vi "Send SCPI Strings.vi"(0 "Resource In":refnum<visa-resource-name>, 1 "Check For SCPI Errors? (T)":bool=TRUE, 5 "SCPI Strings (no term char)":string[](array[string]), 7 "Term Char (0xA)":u8=10 format="%02x", 9 "Num Bytes To Read (256)":u32=256, 11 "error in (no error)":errorcluster, 14 "Trim End Whitespace? (T)":bool=TRUE) -> (4 "Resource Out (dupl)":refnum<visa-resource-name>, 6 "Query Responses":string[](array[string]), 8 "Num Strings Sent":i32, 15 "error out":errorcluster)   [LabVIEW 2009, in "Keithley 622x.lvlib"]
uses:
  Keithley 622x.lvlib
  <vilib>/Utility/error.llb/whitespace.ctl
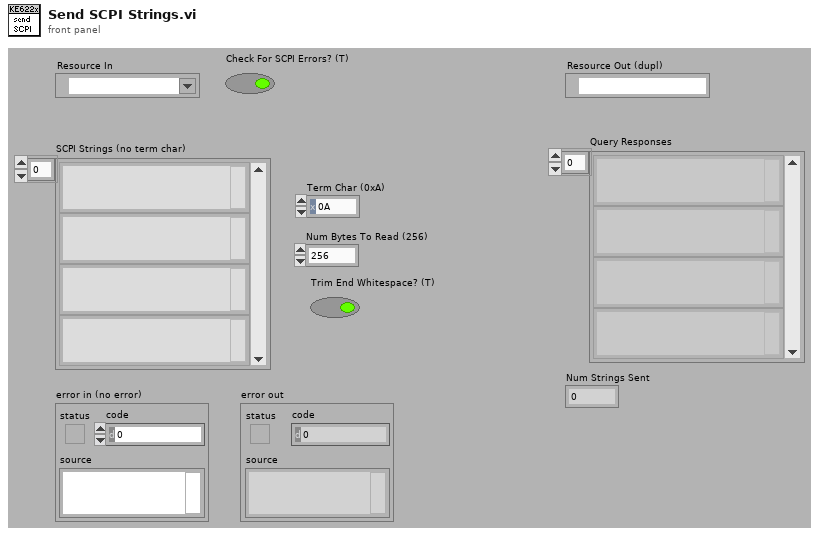
[diagram p1: front panel]
types:
  T1 = typedef "whitespace.ctl" = u16
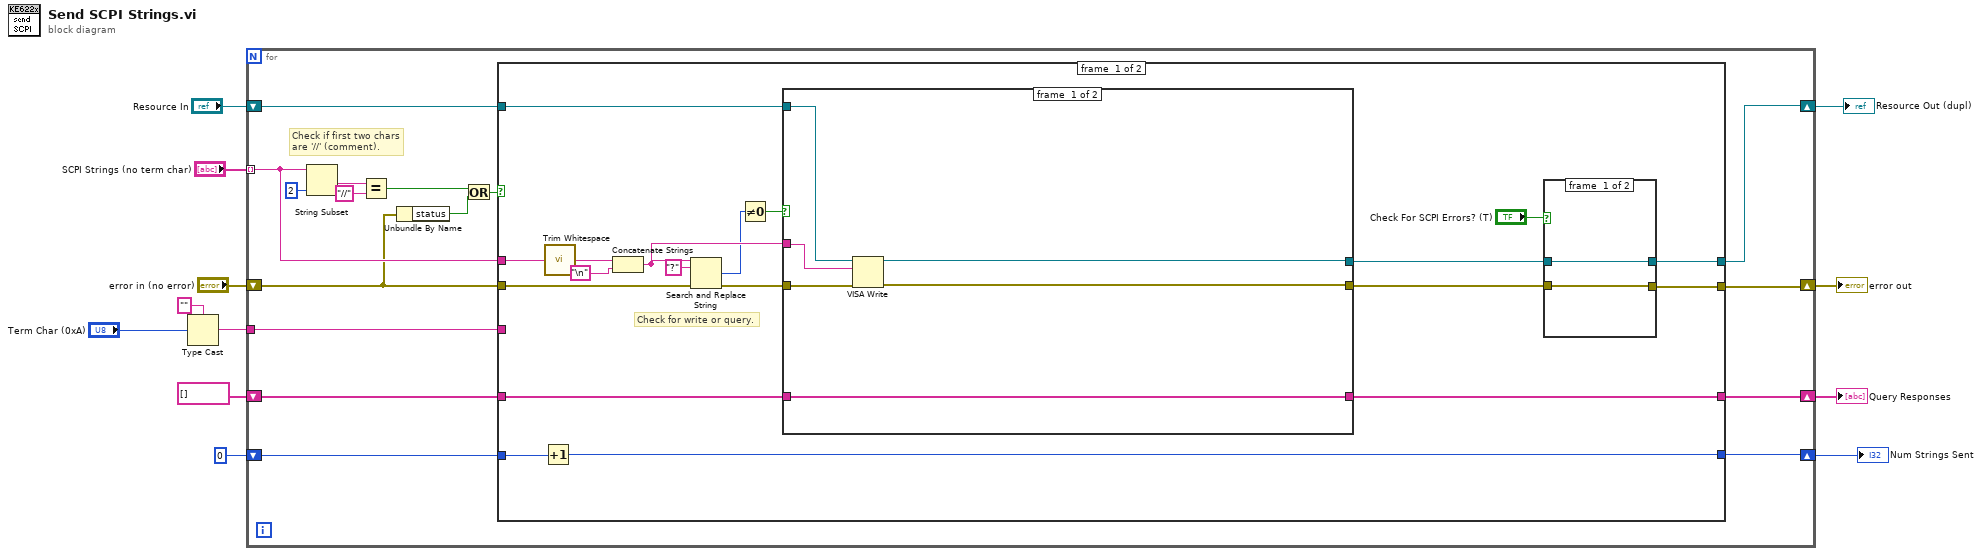
[diagram p0: block diagram]
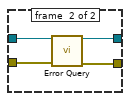
[diagram p2: hidden frame]
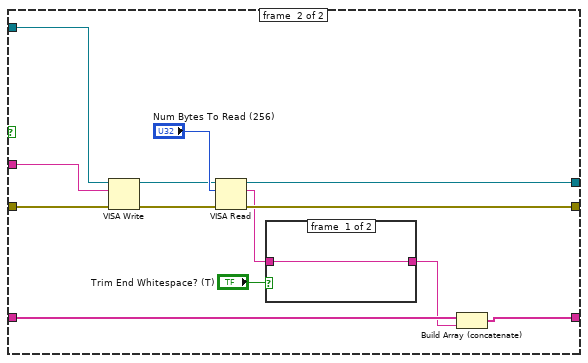
[diagram p3: hidden frame]
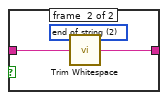
[diagram p4: hidden frame]
diagram:
  n1 = Type Cast(type="", x="Term Char (0xA)") -> (*(type *) &x=w1:string)
  n2 = for {
    tunnel: "SCPI Strings (no term char)" -> [w24] mode=indexing
    shift-right: [w19] -> w6
    shift-left: "error in (no error)" -> [w17]
    shift-right: [w18] -> w5
    shift-left: "Resource In" -> [w23]
    tunnel: w1 -> [w22]
    shift-right: [w20] -> w4
    shift-left: string[] [] -> [w21]
    shift-right: [w13] -> w2
    shift-left: 0 -> [w14]
    # "Check if first two chars\nare '//' (comment)."
    n3 = String Subset(string=w24, length (rest)=2 ("length (rest)")) -> (substring=w27:string)  [unwired: 1 in]
    n4 = Equal?(x=w27, y="//") -> (x = y?=w25:bool)
    n5 = Unbundle By Name(w17) -> ("status"=w15:bool)
    n6 = Or(x=w25, y=w15) -> (x .or. y?=w16:bool)
    n7 = case shown="False" w16 {
      tunnel: w17 -> [w47 w79]
      tunnel: w24 -> [w46 _]
      tunnel: w23 -> [w42 w78]
      tunnel: w22 -> [_ _]
      tunnel: w21 -> [w40 w80]
      tunnel: [w39 w80] -> w20
      tunnel: [w35 w79] -> w19
      tunnel: [w34 w78] -> w18
      tunnel: w14 -> [w33 w77]
      tunnel: [w32 w77] -> w13
      frame #0 {
        # "Check for write or query."
        n8 = Increment(x=w33) -> (x+1=w32:i32)
        n9 = call <vilib>:"Trim Whitespace.vi"("string"=w46) -> ("trimmed string"=w31:string)  [unwired: 1 in]
        n10 = Concatenate Strings(w31, "\n") -> (w41:string)
        n11 = Search and Replace String(input string=w41, search string="?", error in=w47) -> (number of replacements=w30:i32, error out=w43:errorcluster)  [unwired: 5 in, 2 out]
        n12 = Not Equal To 0?(x=w30) -> (x != 0?=w44:bool)
        n13 = case shown="False" w44 {
          tunnel: w43 -> [w58 w72]
          tunnel: w42 -> [w56 w71]
          tunnel: w41 -> [w57 w70]
          tunnel: [w54 w66] -> w37
          tunnel: [w55 w65] -> w36
          tunnel: w40 -> [w59 w62]
          tunnel: [w59 w60] -> w39
          frame #0 {
            n14 = VISA Write(VISA resource name=w56, write buffer=w57, error in (no error)=w58) -> (VISA resource name out=w54:refnum<visa-resource-name>, error out=w55:errorcluster)  [unwired: 1 out]
          }
          frame #1 {
            n15 = VISA Write(VISA resource name=w71, write buffer=w70, error in (no error)=w72) -> (VISA resource name out=w68:refnum<visa-resource-name>, error out=w67:errorcluster)  [unwired: 1 out]
            n16 = VISA Read(VISA resource name=w68, byte count="Num Bytes To Read (256)", error in (no error)=w67) -> (VISA resource name out=w66:refnum<visa-resource-name>, read buffer=w63:string, error out=w65:errorcluster)  [unwired: 1 out]
            n17 = case shown="False" "Trim End Whitespace? (T)" {
              tunnel: w63 -> [w73 w75]
              tunnel: [w73 w74] -> w61
              frame #0 {
              }
              frame #1 {
                w76 = T1 2 items=["both", "start of string", "end of string"] ("location (both)")
                n18 = call <vilib>:"Trim Whitespace.vi"("string"=w75, "location (both)"=w76) -> ("trimmed string"=w74:string)
              }
            }
            n19 = Build Array (concatenate)(w62, w61) -> (w60:string[])
          }
        }
        n20 = case shown="True" "Check For SCPI Errors? (T)" {
          tunnel: w37 -> [w49 w53]
          tunnel: w36 -> [w48 w52]
          tunnel: [w48 w51] -> w35
          tunnel: [w49 w50] -> w34
          frame #0 {
          }
          frame #1 {
            n21 = call "Error Query.vi"("VISA Resource In"=w53, "error in (no error)"=w52) -> ("VISA Resource Out (dupl)"=w50:refnum<visa-resource-name>, "error out"=w51:errorcluster)  [unwired: 10 in, 2 out]
          }
        }
      }
      frame #1 {
        # "Comment (or commented out), or error, so don't do anything."
      }
    }
  }
  "Resource Out (dupl)" <- w5
  "error out" <- w6
  "Query Responses" <- w4
  "Num Strings Sent" <- w2
